vi "v2.4.vi"() -> ()   [LabVIEW 2018]
uses:
  <vilib>/DAQmx/read.llb/DAQmx Read (Analog 1D DBL NChan 1Samp).vi
  <vilib>/DAQmx/create/channels.llb/DAQmx Create Channel (AI-Temperature-Thermocouple).vi
  <vilib>/DAQmx/configure/timing.llb/DAQmx Timing (Sample Clock).vi
  <vilib>/DAQmx/miscellaneous.llb/DAQmx Fill In Error Info.vi
panel:
  in  "Flowrate Control":dbl
  out "Status":T1(ring)
  in  "Stop":bool
  in  "OK Button":bool
  in  "DAQ Properties":cluster{"Sample Rate":dbl}={"Sample Rate"=1.0} {"Sample Rate" min=1.0 max=10000.0 step=1.0}
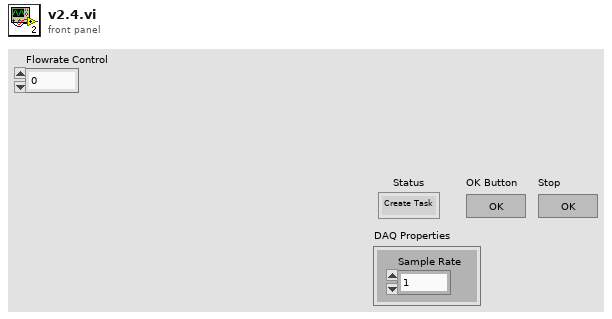
[diagram p1: front panel]
types:
  T1 = enum16{"Create Task", "Change Settings", "Check Settings", "Read Data", "End Task"}
  T2 = enum8{"Enabled", "Disabled", "Disabled and Grayed Out"}
  T3 = cluster{"Line Number":dbl, "Temperature":dbl, "Pressure":dbl, "Flowrate":dbl}[]
  T4 = cluster{"BRNR FC":dbl, "BRNR Nozzle":dbl, "Lance Tip":dbl, "Tube 2 Tmp":dbl, "Tube Tmp":dbl, "GA GAS Tmp":dbl, "Chamber External Temp":dbl}
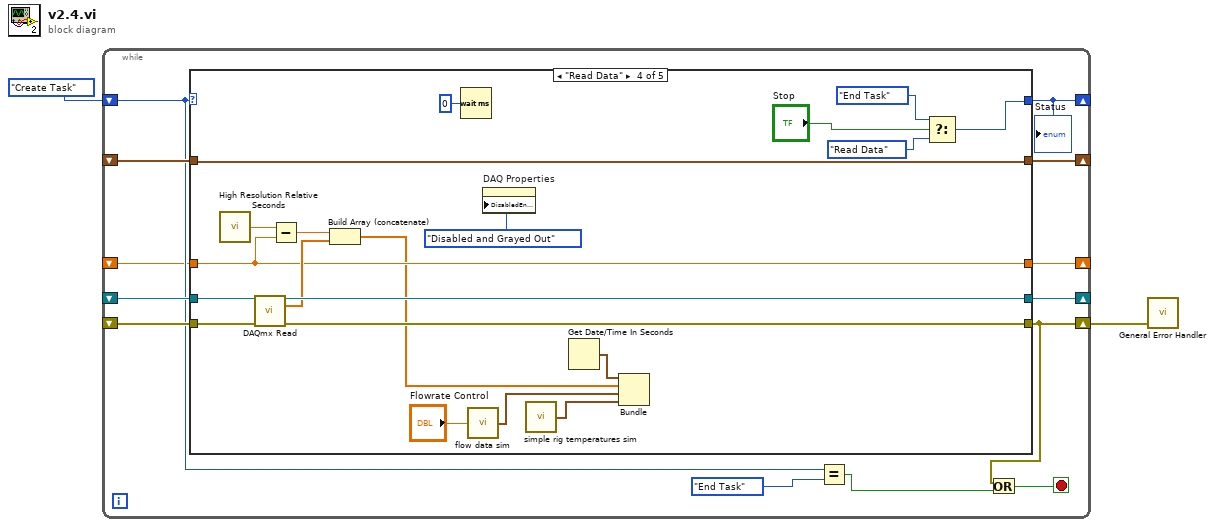
[diagram p0: block diagram]
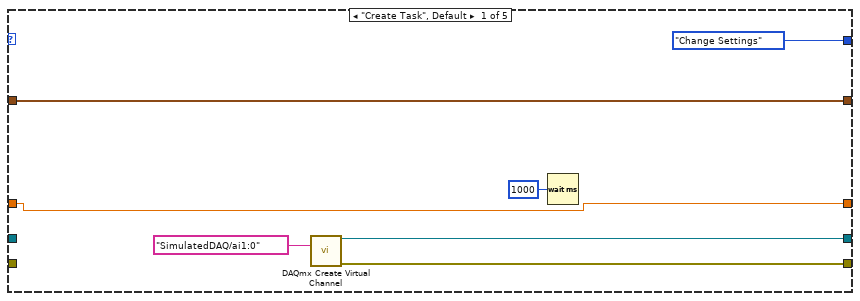
[diagram p2: hidden frame]
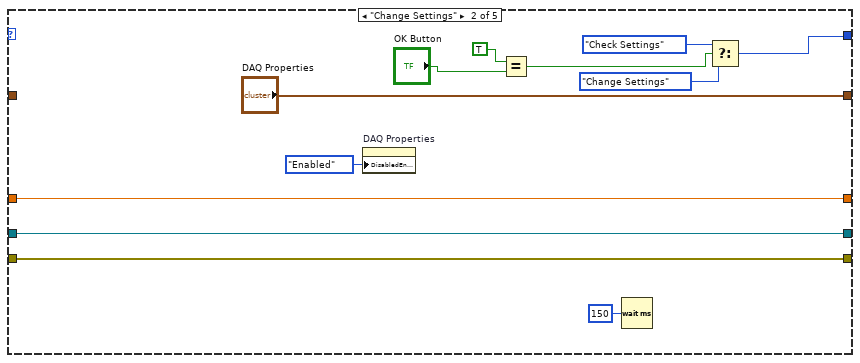
[diagram p3: hidden frame]
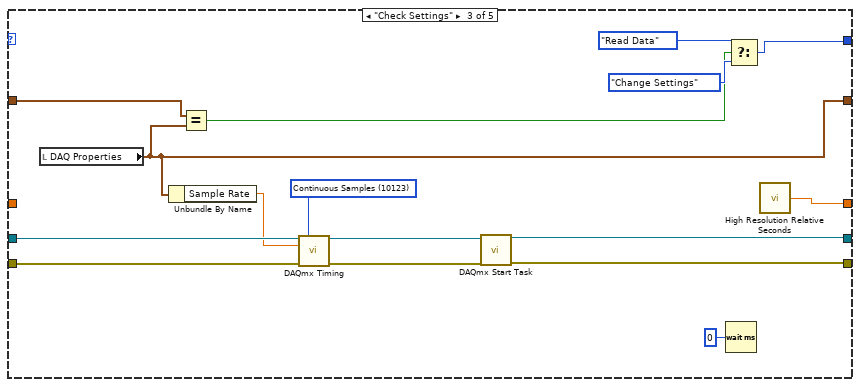
[diagram p4: hidden frame]
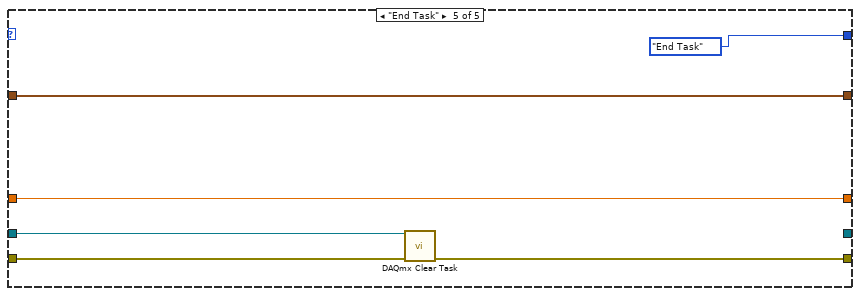
[diagram p5: hidden frame]
diagram:
  n1 = while {
    shift-right: [w10] -> _
    shift-left: T1."Create Task" -> [w5]
    shift-right: [w15] -> _
    shift-left: _ -> [w13]
    shift-right: [w9] -> w1
    shift-left: _ -> [w12]
    shift-right: [w14] -> _
    shift-left: _ -> [w11]
    shift-right: [w4] -> _
    shift-left: _ -> [w3]
    stop <- w8 stop-if-true
    n2 = case shown="\"Read Data\"" w5 {
      tunnel: [w22 w34 w39 w67 _] -> w15
      tunnel: [w21 w33 w38 w66 w76] -> w9
      tunnel: [T1."Change Settings" w27 w46 w64 T1."End Task"] -> w10
      tunnel: [w18 "DAQ Properties" w42 w68 w75] -> w14
      tunnel: w13 -> [_ w34 w45 w70 w73]
      tunnel: w12 -> [_ w33 w44 w69 w72]
      tunnel: w11 -> [w18 _ w50 w68 w75]
      tunnel: [w16 w24 w35 w57 w71] -> w4
      tunnel: w3 -> [w16 w24 _ w57 w71]
      frame "Create Task", Default {
        n3 = call-poly <vilib>:"DAQmx Create Virtual Channel.vi"("physical channels"=tag "SimulatedDAQ/ai1:0") -> ("task out"=w22:refnum<k21>, "error out"=w21:errorcluster)  [unwired: 13 in]
        n4 = Wait (ms)(milliseconds to wait=u32 1000) -> ()  [unwired: 1 out]
      }
      frame "Change Settings" {
        n5 = property on="DAQ Properties" class="Clust (strict)"("DisabledEnum"=T2."Enabled" ("Disabled")) -> ()  [unwired: 2 in, 2 out]
        n6 = Equal?(x=TRUE, y="OK Button") -> (x = y?=w29:bool)
        n7 = Wait (ms)(milliseconds to wait=u32 150) -> ()  [unwired: 1 out]
        n8 = Select(t=T1."Check Settings", s=w29, f=T1."Change Settings") -> (s? t:f=w27:T1)
      }
      frame "Check Settings" {
        w36 = 10123 items=["Finite Samples"=10178, "Continuous Samples"=10123, "Hardware Timed Single Point"=12522] ("sample mode")
        n9 = local read "DAQ Properties"() -> (w42:cluster{"Sample Rate":dbl})
        n10 = Unbundle By Name(w42) -> ("Sample Rate"=w43:dbl)
        n11 = Equal?(x=w50, y=w42) -> (x = y?=w37:bool)
        n12 = call-poly <vilib>:"DAQmx Timing.vi"("task/channels in"=w45, "sample mode"=w36, "rate"=w43, "error in"=w44) -> ("task out"=w41:refnum<k21>, "error out"=w40:errorcluster)  [unwired: 10 in]
        n13 = call <vilib>:"DAQmx Start Task.vi"("task/channels in"=w41, "error in"=w40) -> ("task out"=w39:refnum<k21>, "error out"=w38:errorcluster)  [unwired: 12 in]
        n14 = Wait (ms)(milliseconds to wait=u32 0) -> ()  [unwired: 1 out]
        n15 = Select(t=T1."Read Data", s=w37, f=T1."Change Settings") -> (s? t:f=w46:T1)
        n16 = call <vilib>:"High Resolution Relative Seconds.vi"() -> ("relative seconds"=w35:dbl)
      }
      frame "Read Data" {
        n17 = call <vilib>:"High Resolution Relative Seconds.vi"() -> ("relative seconds"=w60:dbl)
        n18 = call-poly <vilib>:"DAQmx Read.vi"("task/channels in"=w70, "error in"=w69) -> ("task out"=w67:refnum<k21>, "data"=w59:dbl[], "error out"=w66:errorcluster)  [unwired: 11 in]
        n19 = Subtract(x=w60, y=w57) -> (x-y=w58:dbl)
        n20 = Build Array (concatenate)(w58, w59) -> (w54:dbl[])
        n21 = Wait (ms)(milliseconds to wait=u32 0) -> ()  [unwired: 1 out]
        n22 = call "flow data sim.vi"("Boondoggle Input"="Flowrate Control") -> ("Flowrate Data"=w53:T3)
        n23 = property on="DAQ Properties" class="Clust (strict)"("DisabledEnum"=T2."Disabled and Grayed Out" ("Disabled")) -> ()  [unwired: 2 in, 2 out]
        n24 = call "simple rig temperatures sim.vi"() -> ("Rig Temperatures"=w51:T4)
        n25 = Get Date/Time In Seconds() -> (seconds since 1Jan1904=w55:timestamp)
        n26 = Bundle("seconds since 1Jan1904"=w55, w54, "Flowrate Data"=w53, "Rig Temperatures"=w51) -> ()  [unwired: 1 in, 1 out]
        n27 = Select(t=T1."End Task", s="Stop", f=T1."Read Data") -> (s? t:f=w64:T1)
      }
      frame "End Task" {
        n28 = call <vilib>:"DAQmx Clear Task.vi"("task in"=w73, "error in"=w72) -> ("error out"=w76:errorcluster)  [unwired: 13 in]
      }
    }
    "Status" <- w10
    n29 = Equal?(x=w5, y=T1."End Task") -> (x = y?=w6:bool)
    n30 = Or(x=w9, y=w6) -> (x .or. y?=w8:bool)
  }
  n31 = call <vilib>:"General Error Handler.vi"("error in (no error)"=w1) -> ()  [unwired: 10 in, 5 out]
